vi "monitorPhotodiode.vi"(8 "error in (no error)":errorcluster, 9 "Photdiode warning in":bool, 10 "Led warning in":bool, 11 "Arduino session":refnum<visa-resource-name>) -> (0 "error out":errorcluster, 1 "Photodiode Warning":bool, 2 "LED Warning":bool, 3 "Arduino session":refnum<visa-resource-name>, 4 "PD Value":i32)   [LabVIEW 2017]
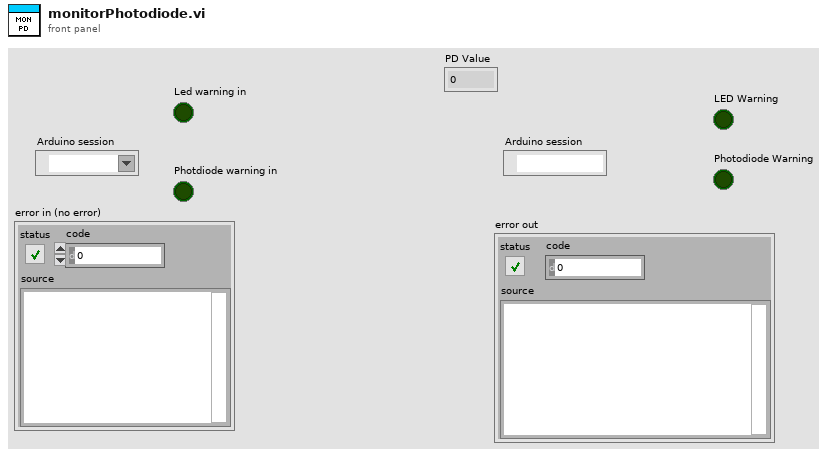
[diagram p1: front panel]
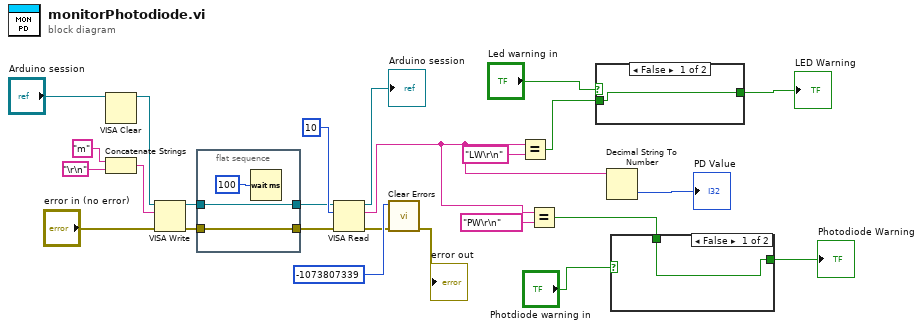
[diagram p0: block diagram]
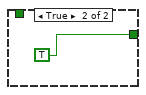
[diagram p2: hidden frame]
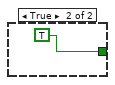
[diagram p3: hidden frame]
diagram:
  n1 = VISA Clear(VISA resource name="Arduino session") -> (VISA resource name out=w14:refnum<visa-resource-name>)  [unwired: 1 in, 1 out]
  n2 = Concatenate Strings("m" ("string"), "\r\n") -> (w19:string)
  n3 = VISA Write(VISA resource name=w14, write buffer=w19, error in (no error)="error in (no error)") -> (VISA resource name out=w20:refnum<visa-resource-name>, error out=w16:errorcluster)  [unwired: 1 out]
  n4 = flat-sequence {
    tunnel: [w27] -> w21
    tunnel: w20 -> [w27]
    tunnel: [w26] -> w17
    tunnel: w16 -> [w26]
    frame #0 {
      n5 = Wait (ms)(milliseconds to wait=u32 100) -> ()  [unwired: 1 out]
    }
  }
  n6 = VISA Read(VISA resource name=w21, byte count=u32 10, error in (no error)=w17) -> (VISA resource name out=→"Arduino session":refnum<visa-resource-name>, read buffer=w2:string, error out=w12:errorcluster)  [unwired: 1 out]
  n7 = call <vilib>:"Clear Errors.vi"("error in (no error)"=w12, "specific error code to clear (0: all)"=-1073807339) -> ("error out"=→"error out":errorcluster)  [unwired: 4 in, 1 out]
  n8 = Equal?(x=w2, y="LW\r\n") -> (x = y?=w7:bool)
  n9 = Equal?(x=w2, y="PW\r\n") -> (x = y?=w3:bool)
  n10 = case shown="False" "Led warning in" {
    tunnel: [w29 TRUE] -> w8
    tunnel: w7 -> [w29 _]
    frame False {
    }
    frame True {
    }
  }
  "LED Warning" <- w8
  n11 = Decimal String To Number(string=w2) -> (number=→"PD Value":i32)  [unwired: 2 in, 1 out]
  n12 = case shown="False" "Photdiode warning in" {
    tunnel: [w31 TRUE] -> w5
    tunnel: w3 -> [w31 _]
    frame False {
    }
    frame True {
    }
  }
  "Photodiode Warning" <- w5
